vi "FFT.vi"() -> ()   [LabVIEW 2021]
uses:
  <vilib>/Analysis/4window.llb/windowTd.ctl
  <vilib>/Analysis/0measdsp.llb/Scaled Time Domain Window (DBL).vi
  <vilib>/express/express analysis/Spectral/Block/exnSpectralBlock spectral measurements peak poly.vi
  <vilib>/express/express analysis/Spectral/Block/exnSpectralBlock spectral measurements peak DDT.vi
  <vilib>/express/express analysis/Spectral/Block/exnSpectralBlock spectral measurements PSD poly.vi
  <vilib>/express/express analysis/Spectral/Block/exnSpectralBlock spectral measurements PSD DDT.vi
  <vilib>/express/express analysis/Spectral/XNode/ExpressSpectralMeasurementsBlockNode.xnode
  <vilib>/Analysis/NI_AALPro.lvlib
panel:
  out "Densidad espectral":dbl[](graph)
  in  "FFT VENTANA":dbl
  in  "window":T1 items=["Rectangle"=0, "Hanning"=1, "Hamming"=2, "Blackman-Harris"=3, "Exact Blackman"=4, "Blackman"=5, "Flat Top"=6, "4 Term B-Harris "=7, "7 Term B-Harris"=8, "Low Sidelobe"=9, "Blackman Nuttall"=11, "Triangle"=30, "Bartlett-Hanning"=31, "Bohman"=32, "Parzen"=33, "Welch"=34, "Kaiser"=60, "Dolph-Chebyshev"=61, "Gaussian"=62]
  in  "Frecuencia":dbl=250.0 caption="Frequency"
  out "FFT EXPRESS":dbl[](graph)
  out "ORIGINAL":dbl[](graph)
  out "FFT VENTANEO":dbl[](graph)
  out "FFT APLICACIÓN":dbl[][](graph)
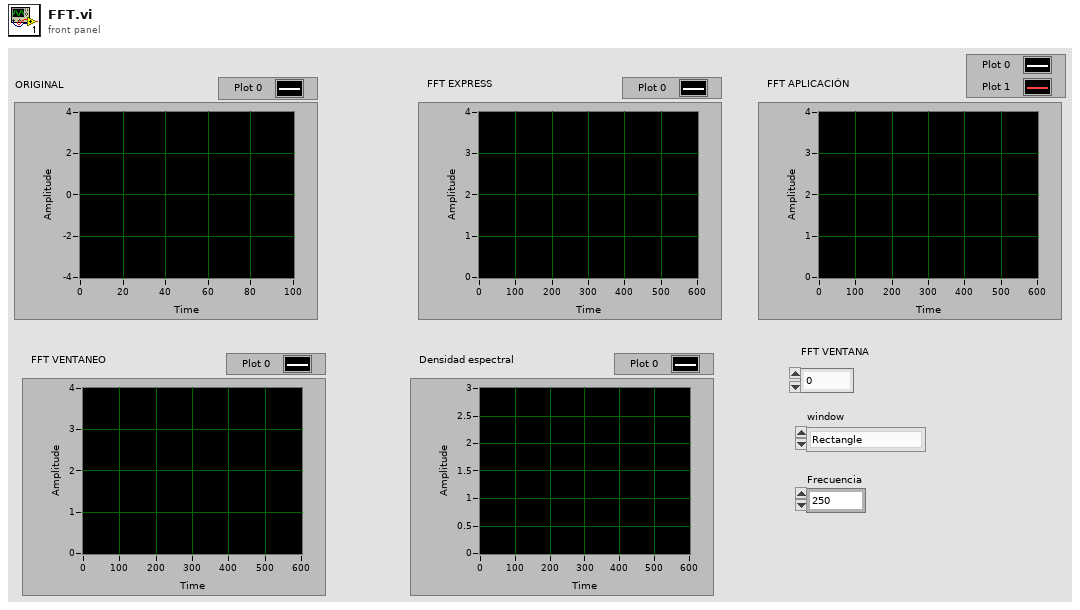
[diagram p1: front panel]
types:
  T1 = typedef "NI_AALPro.lvlib/windowTd.ctl" = u32
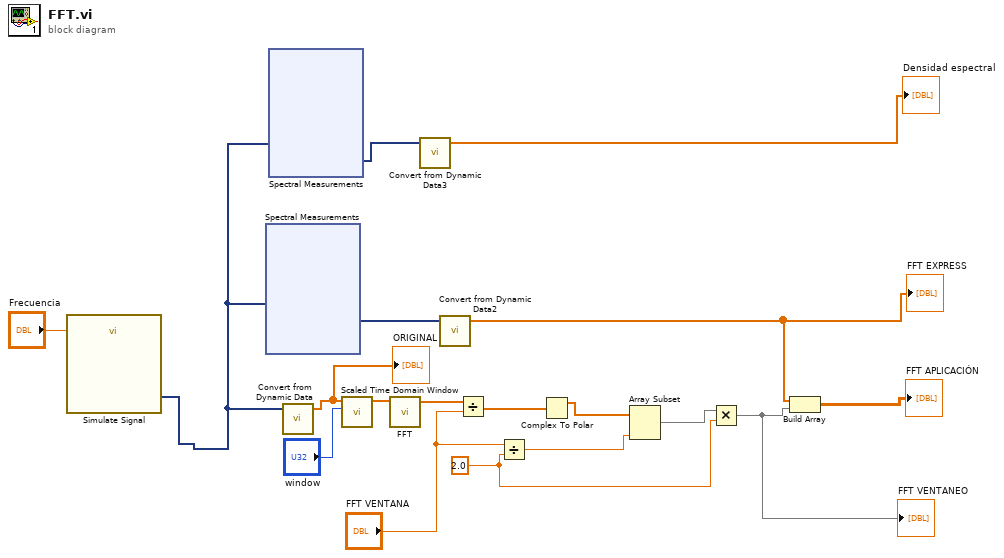
[diagram p0: block diagram]
diagram:
  w10 = 2.0 ("y")
  n1 = call "Simulate Signal"("Frequency"="Frecuencia") -> ("Sine"=w1:dynamicdata)  [unwired: 13 in, 1 out]
  n2 = xnode "Spectral Measurements"("Signals"=w1) -> ("FFT - (Peak)"=w8:dynamicdata)  [unwired: 1 in, 2 out]
  n3 = xnode "Spectral Measurements"("Signals"=w1) -> ("PSD"=w3:dynamicdata)  [unwired: 1 in, 1 out]
  n4 = call "Convert from Dynamic Data"("Dynamic Data Type"=w1) -> ("Array"=w7:dbl[])  [unwired: 3 in]
  "ORIGINAL" <- w7
  n5 = call-poly <vilib>:"Scaled Time Domain Window.vi"("window"="window", "X"=w7) -> ("Windowed X"=w18:dbl[])  [unwired: 7 in, 2 out]
  n6 = call-poly <vilib>:"FFT.vi"("X"=w18) -> ("FFT {X}"=w15:cdb[])  [unwired: 9 in, 1 out]
  n7 = call "Convert from Dynamic Data3"("Dynamic Data Type"=w3) -> ("Array"=→"Densidad espectral":dbl[])  [unwired: 3 in]
  n8 = call "Convert from Dynamic Data2"("Dynamic Data Type"=w8) -> ("Array"=w5:dbl[])  [unwired: 3 in]
  "FFT EXPRESS" <- w5
  n9 = Divide(x=w15, y="FFT VENTANA") -> (x/y=w13:cdb[])
  n10 = Divide(x="FFT VENTANA", y=w10) -> (x/y=w11:dbl)
  n11 = Complex To Polar(r * e^(i*theta)=w13) -> (r=w12:dbl[])  [unwired: 1 out]
  n12 = Array Subset(array=w12, length=w11) -> (w9:dbl[])  [unwired: 1 in]
  n13 = Multiply(x=w9, y=w10) -> (x*y=w4:dbl[])
  "FFT VENTANEO" <- w4
  n14 = Build Array(w5, w4) -> (→"FFT APLICACIÓN":dbl[][])
